vi "Configure.vi"(8 "error in (no error)":errorcluster, 9 "Record":bool=TRUE, 10 "Recording Channels":refnum<k21>="All4498", 11 "Electrophysiology in":refnum<class "Electrophysiology.lvclass">) -> (0 "error out":errorcluster, 3 "Electrophysiology out":refnum<class "Electrophysiology.lvclass">)   [LabVIEW 2012, in "AcquisitionCoreObjects.lvlib" / "Electrophysiology.lvclass"]
uses:
  Electrophysiology.lvclass
  AcquireTraces/AcquireTraces.lvclass
  <vilib>/sound2/lvsound2.llb/Sampling Mode.ctl
  <vilib>/sound2/lvsound2.llb/Sound Data Format.ctl
  Electrophysiology.lvclass/Electrophysiology.ctl
  <resource>/objmgr/daqmx.rc
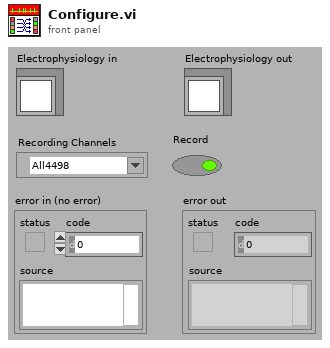
[diagram p1: front panel]
types:
  T1 = typedef "Sound Data Format.ctl" = cluster{"sample rate (S/s)":dbl, "number of channels":i32, "bits per sample":i32}
  T2 = typedef "Sampling Mode.ctl" = i32
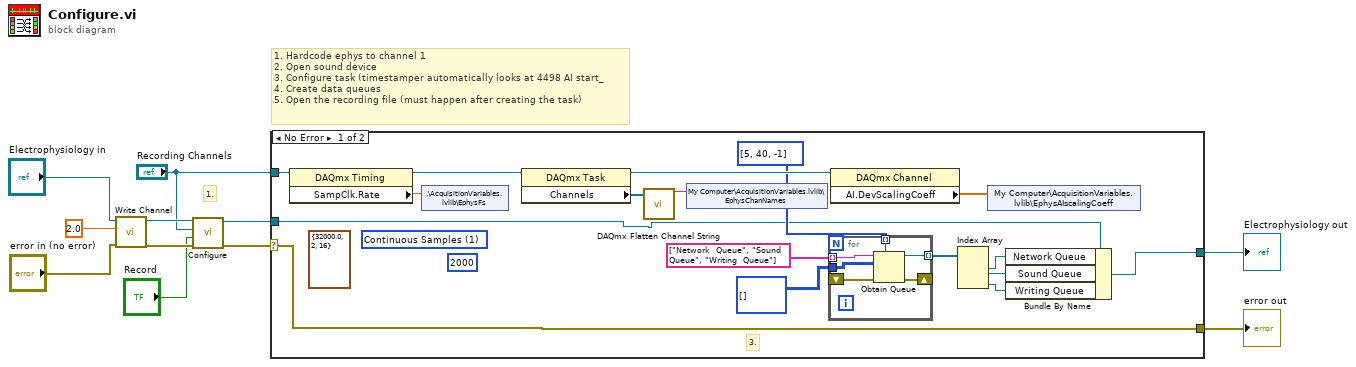
[diagram p0: block diagram]
diagram:
  # "1."
  # "1. Hardcode ephys to channel 1\n2. Open sound device\n3. Configure task (timestamper automatically looks at 4498 AI start_\n4. Create data queues\n5. Open the recording file (must happen after creating the task)"
  n1 = call-dynamic "Write Channel.vi"("error in (no error)"="error in (no error)", "Channel"=2.0, "AcquistionObject in"="Electrophysiology in") -> ("error out"=w3:errorcluster, "AcquistionObject out"=w4:refnum<class "Electrophysiology.lvclass">)  [unwired: 7 in]
  n2 = call-parent "Configure.vi"("error in (no error)"=w3, "Record"="Record", "Recording Channels"="Recording Channels", "AcquireTraces in"=w4) -> ("error out"=w8:errorcluster, "AcquireTraces out"=w9:refnum<class "Electrophysiology.lvclass">)  [unwired: 6 in]
  n3 = case shown="No Error" w8 {
    selector: w8 -> [w13 w36]
    tunnel: [w13 w36] -> w11
    tunnel: [w22 w35] -> w10
    tunnel: w9 -> [w12 w35]
    tunnel: "Recording Channels" -> [w21 _]
    frame No Error {
      (unwired) T1 {"sample rate (S/s)"=32000.0, "number of channels"=2, "bits per sample"=16} ("sound format")
      (unwired) 2000 ("number of samples/ch")
      (unwired) T2 1 items=["Finite Samples", "Continuous Samples"] ("sample mode")
      # "3."
      n4 = property class="DAQmx Timing"(reference=w21) -> (reference out=w20:refnum<k21>, "SampClk.Rate"=w19:dbl)  [unwired: 1 in, 1 out]
      n5 = shared-variable ".\\AcquisitionVariables.lvlib\\EphysFs"(w19) -> ()  [unwired: 1 in, 1 out]
      n6 = property class="DAQmx Task"(reference=w20) -> (reference out=w16:refnum<k21>, "Channels"=w18:refnum<k21>[])  [unwired: 1 in, 1 out]
      n7 = call <vilib>:"DAQmx Flatten Channel String.vi"("names in"=w18) -> ("names out"=w17:string)  [unwired: 13 in, 1 out]
      n8 = shared-variable "My Computer\\AcquisitionVariables.lvlib\\EphysChanNames"(w17) -> ()  [unwired: 1 in, 1 out]
      n9 = for {
        tunnel: string[] ["Network  Queue", "Sound  Queue", "Writing  Queue"] -> [w34] mode=indexing
        tunnel: i32[][] [] -> [w33]
        tunnel: [w32] -> w26 mode=indexing
        shift-right: [w31] -> _
        shift-left: _ -> [w30]
        tunnel: i32[] [5, 40, -1] -> [w29] mode=indexing
        n10 = Obtain Queue(max queue size (-1, unlimited)=w29, name (unnamed)=w34, element data type=w33, error in (no error)=w30) -> (queue out=w32:refnum<queue>, error out=w31:errorcluster)  [unwired: 1 in, 1 out]
      }
      n11 = property class="DAQmx Channel"(reference=w16) -> ("AI.DevScalingCoeff"=w15:dbl[])  [unwired: 1 in, 2 out]
      n12 = Index Array(array=w26) -> (element #1=w25:refnum<queue>, element #2=w24:refnum<queue>, element #3=w23:refnum<queue>)  [unwired: 3 in]
      n13 = shared-variable "My Computer\\AcquisitionVariables.lvlib\\EphysAIscalingCoeff"(w15) -> ()  [unwired: 1 in, 1 out]
      n14 = Bundle By Name(cluster=w12, "Network Queue"=w25, "Sound Queue"=w24, "Writing Queue"=w23) -> (w22:refnum<class "Electrophysiology.lvclass">)
    }
    frame Error {
    }
  }
  "error out" <- w11
  "Electrophysiology out" <- w10
